vi "Subvi identifier.vi"(11 "BrickReference in":T1) -> (3 "Array":dbl[](array[numeric]))   [LabVIEW 2016]
uses:
  <vilib>/NXT/Subs/LVHSConnector.ctl
  <vilib>/NXT/LegoClasses/BrickReference/BrickReference.lvclass
  <vilib>/NXT/Block Support/NXT_InputPort.ctl
  <vilib>/NXT/Dual Mode Library/Sensors/Touch_Pressed.vi
  <vilib>/NXT/Dual Mode Library/Sensors/EV3_Color_RGB.vi
  <vilib>/NXT/Dual Mode Library/prims/inRangeAndCoerce/inRangeAndCoerce_int.vi
  <vilib>/NXT/Dual Mode Library/Sensors/EV3_Color_Color.vi
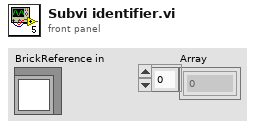
[diagram p1: front panel]
types:
  T1 = typedef "LVHSConnector.ctl" = refnum<class "BrickReference.lvclass">
  T2 = typedef "NXT_InputPort.ctl" = u32
  T3 = typedef "ColorSensorColors.ctl" = enum16{"No Color", "Black", "Blue", "Green", "Yellow", "Red", "White", "Brown"}
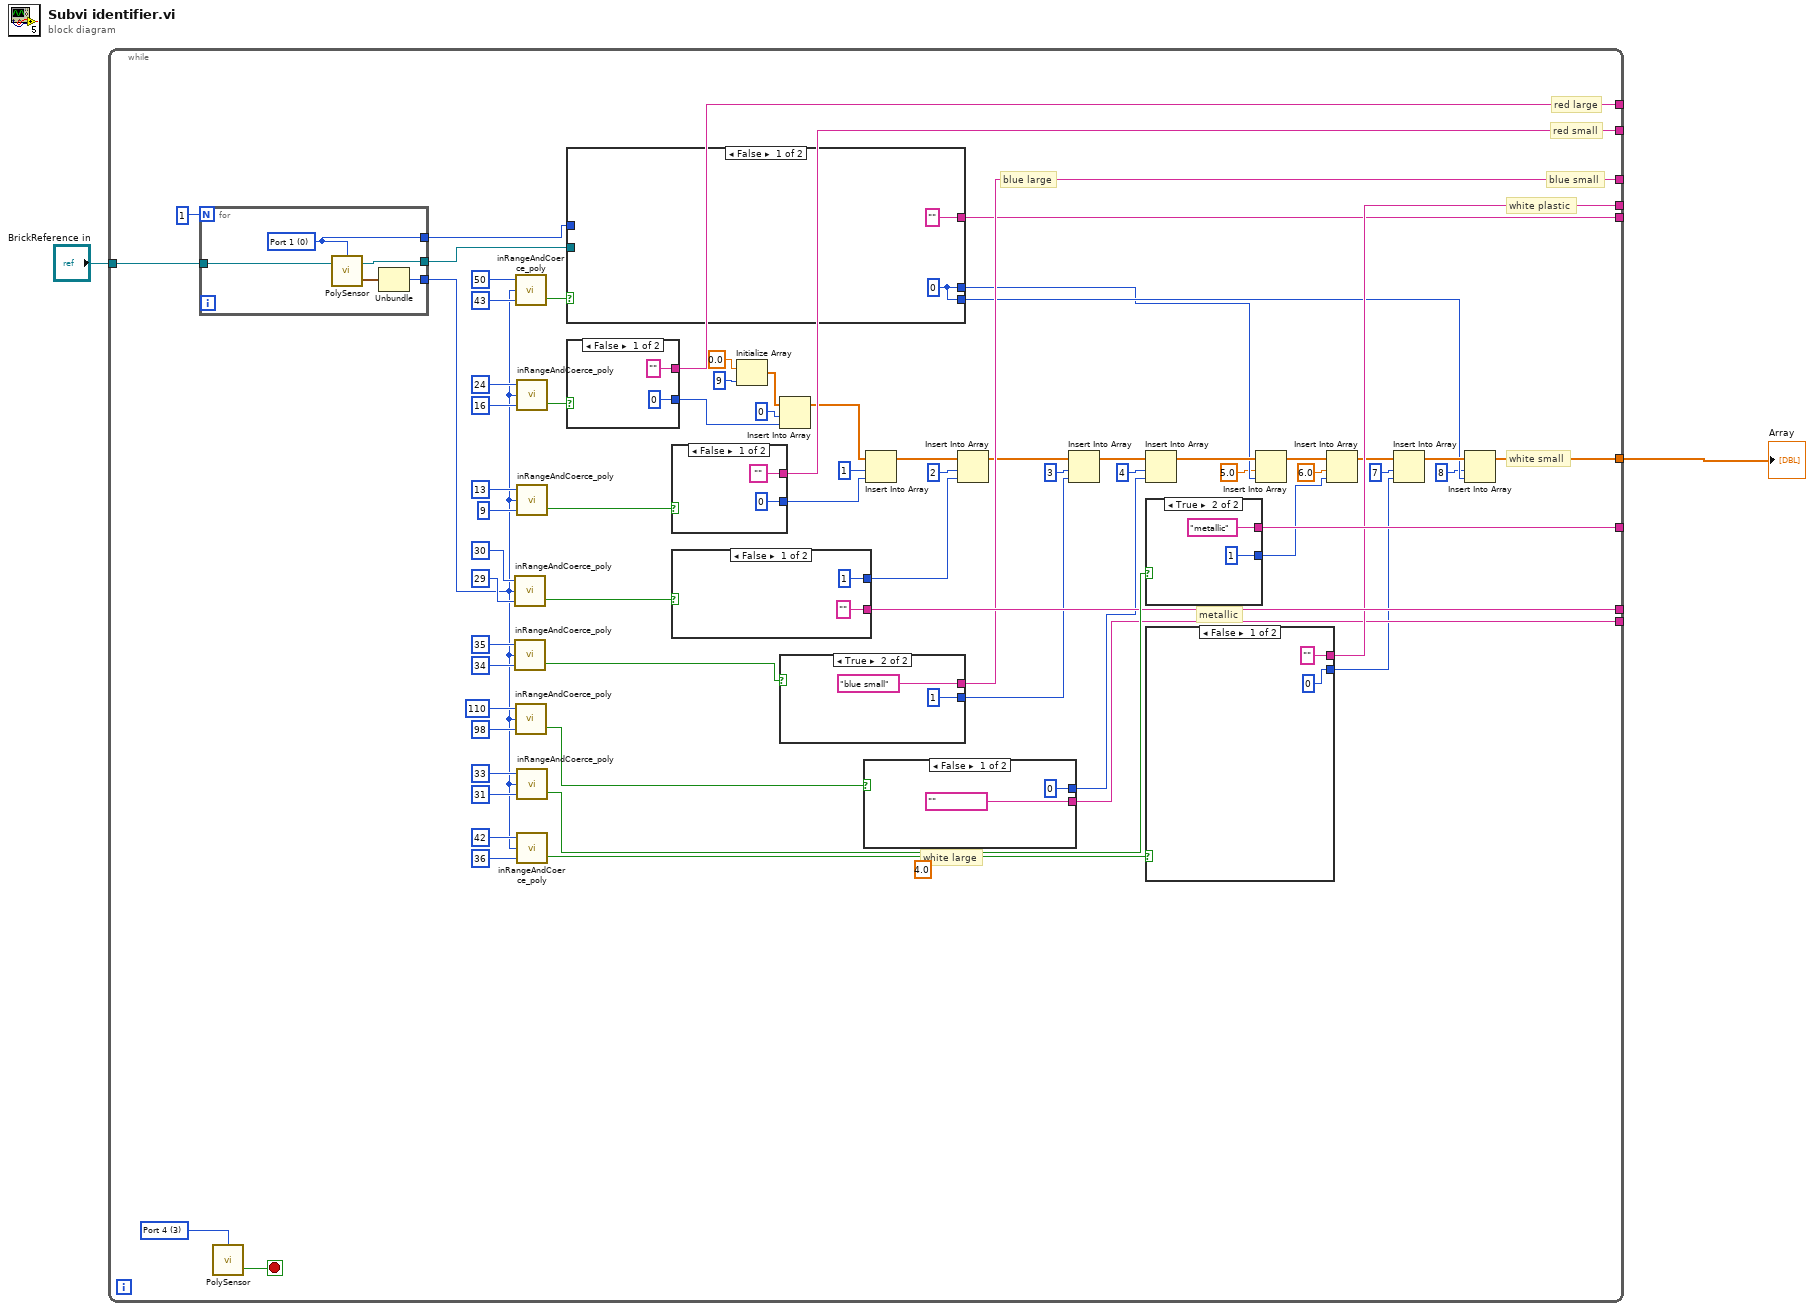
[diagram p0: block diagram]
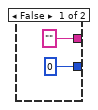
[diagram p2: hidden frame]
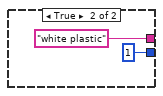
[diagram p3: hidden frame]
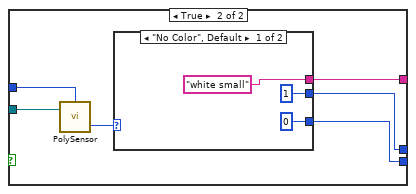
[diagram p4: hidden frame]
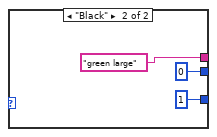
[diagram p5: hidden frame]
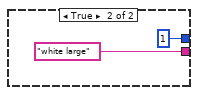
[diagram p6: hidden frame]
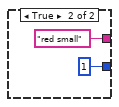
[diagram p7: hidden frame]
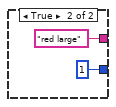
[diagram p8: hidden frame]
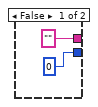
[diagram p9: hidden frame]
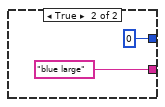
[diagram p10: hidden frame]
diagram:
  n1 = while {
    tunnel: "BrickReference in" -> [w47]
    tunnel: [w41] -> _
    tunnel: [w40] -> _
    tunnel: [w39] -> _
    tunnel: [w38] -> _
    tunnel: [w37] -> _
    tunnel: [w36] -> _
    tunnel: [w35] -> _
    tunnel: [w34] -> _
    tunnel: [w3] -> w2
    stop <- w50 stop-if-true
    (unwired) sgl 4.0 ("Time (1 sec)")
    w49 = T2 3 items=["Port 1", "Port 2", "Port 3", "Port 4"] ("Port (Port 1)")
    # "metallic"
    # "white plastic"
    # "white small"
    # "white large"
    # "red small"
    # "red large"
    # "blue small"
    # "blue large"
    n2 = for {
      N: 1 -> [_]
      tunnel: w47 -> [w75]
      tunnel: [w74] -> w43
      tunnel: [w73] -> w33
      tunnel: [w72] -> w42
      w72 = T2 0 items=["Port 1", "Port 2", "Port 3", "Port 4"] ("Port (Port 1)")
      n3 = call-poly <vilib>:"PolySensor.vi"("NXT/EV3"=w75, "Port (Port 1)"=w72) -> ("RGB Color"=w76:cluster{"Red":u8, "Green":u8, "Blue":u8}, "NXT/EV3"=w73:T1)  [unwired: 1 in]
      n4 = Unbundle(w76) -> ("Green"=w74:u8)  [unwired: 2 out]
    }
    n5 = call-poly <vilib>:"PolySensor.vi"("Port (Port 1)"=w49) -> ("Yes / No"=w50:bool)  [unwired: 2 in, 1 out]
    n6 = call-poly <vilib>:"inRangeAndCoerce_poly.vi"("lower limit"=29, "x"=w43, "upper limit"=30) -> ("In Range?"=w58:bool)  [unwired: 1 out]
    n7 = call-poly <vilib>:"inRangeAndCoerce_poly.vi"("lower limit"=34, "x"=w43, "upper limit"=35) -> ("In Range?"=w57:bool)  [unwired: 1 out]
    n8 = call-poly <vilib>:"inRangeAndCoerce_poly.vi"("lower limit"=43, "x"=w43, "upper limit"=50) -> ("In Range?"=w53:bool)  [unwired: 1 out]
    n9 = call-poly <vilib>:"inRangeAndCoerce_poly.vi"("lower limit"=98, "x"=w43, "upper limit"=110) -> ("In Range?"=w54:bool)  [unwired: 1 out]
    n10 = call-poly <vilib>:"inRangeAndCoerce_poly.vi"("lower limit"=16, "x"=w43, "upper limit"=24) -> ("In Range?"=w56:bool)  [unwired: 1 out]
    n11 = call-poly <vilib>:"inRangeAndCoerce_poly.vi"("lower limit"=9, "x"=w43, "upper limit"=13) -> ("In Range?"=w55:bool)  [unwired: 1 out]
    n12 = call-poly <vilib>:"inRangeAndCoerce_poly.vi"("lower limit"=31, "x"=w43, "upper limit"=33) -> ("In Range?"=w44:bool)  [unwired: 1 out]
    n13 = call-poly <vilib>:"inRangeAndCoerce_poly.vi"("lower limit"=36, "x"=w43, "upper limit"=42) -> ("In Range?"=w52:bool)  [unwired: 1 out]
    n14 = case shown="False" w53 {
      tunnel: ["" w90] -> w35
      tunnel: w42 -> [_ w92]
      tunnel: w33 -> [_ w89]
      tunnel: [w85 w88] -> w5
      tunnel: [w85 w87] -> w12
      frame False {
        w85 = 0
      }
      frame True {
        n15 = call-poly <vilib>:"PolySensor.vi"("NXT/EV3"=w89, "Port (Port 1)"=w92) -> ("Detected Color"=w91:T3)  [unwired: 1 in, 1 out]
        n16 = case shown="\"No Color\", Default" w91 {
          tunnel: ["white small" "green large"] -> w90
          tunnel: [1 0] -> w88
          tunnel: [0 1] -> w87
          frame "No Color", Default {
          }
          frame "Black" {
          }
        }
      }
    }
    n17 = case shown="False" w56 {
      tunnel: ["" "red large"] -> w39
      tunnel: [0 1] -> w29
      frame False {
      }
      frame True {
      }
    }
    n18 = case shown="False" w55 {
      tunnel: ["" "red small"] -> w38
      tunnel: [0 1] -> w23
      frame False {
      }
      frame True {
      }
    }
    n19 = case shown="False" w58 {
      tunnel: ["" "blue large"] -> w41
      tunnel: [1 0] -> w24
      frame False {
      }
      frame True {
      }
    }
    n20 = Initialize Array(0.0 ("element"), 9 ("dimension size")) -> (w22:dbl[])
    n21 = Insert Into Array(array=w22, index=0, new element=w29) -> (w21:dbl[])
    n22 = case shown="True" w57 {
      tunnel: ["" "blue small"] -> w40
      tunnel: [0 1] -> w28
      frame False {
      }
      frame True {
      }
    }
    n23 = case shown="False" w54 {
      tunnel: ["" "white large"] -> w34
      tunnel: [0 1] -> w14
      frame False {
      }
      frame True {
      }
    }
    n24 = Insert Into Array(array=w21, index=1, new element=w23) -> (w20:dbl[])
    n25 = Insert Into Array(array=w20, index=2, new element=w24) -> (w19:dbl[])
    n26 = Insert Into Array(array=w19, index=3, new element=w28) -> (w18:dbl[])
    n27 = Insert Into Array(array=w18, index=4, new element=w14) -> (w8:dbl[])
    n28 = case shown="True" w44 {
      tunnel: ["" "metallic"] -> w37
      tunnel: [0 1] -> w6
      frame False {
      }
      frame True {
      }
    }
    n29 = case shown="False" w52 {
      tunnel: ["" "white plastic"] -> w36
      tunnel: [0 1] -> w11
      frame False {
      }
      frame True {
      }
    }
    n30 = Insert Into Array(array=w8, index=5.0 ("new element/subarray"), new element=w5) -> (w17:dbl[])
    n31 = Insert Into Array(array=w17, index=6.0 ("new element/subarray"), new element=w6) -> (w16:dbl[])
    n32 = Insert Into Array(array=w16, index=7, new element=w11) -> (w15:dbl[])
    n33 = Insert Into Array(array=w15, index=8, new element=w12) -> (w3:dbl[])
  }
  "Array" <- w2
